vi "Word Wrapping in Picture Control.vi"() -> ()   [LabVIEW 2023]
doc: "This VI takes an array of strings and fades the text in and out of a 2D Picture."
panel:
  in  "Text orientation":T1(ring)
  in  "Text":string[](array[string])=["Demonstrates the use of", "the Draw Text at Point VI", "to draw animated text", "within a 2D Picture."]
  in  "Stop":bool
  out "Picture":picture
  # "Overview: Demonstrates the use of the Draw Text at Point VI to draw animated text within a 2D Picture.\nInstructions: \n1. Run the VI. \n2. Change the Text and Text Orientation values to modify the appearance of the animated text in the Picture indicator.\n3. Click Stop to stop the VI."
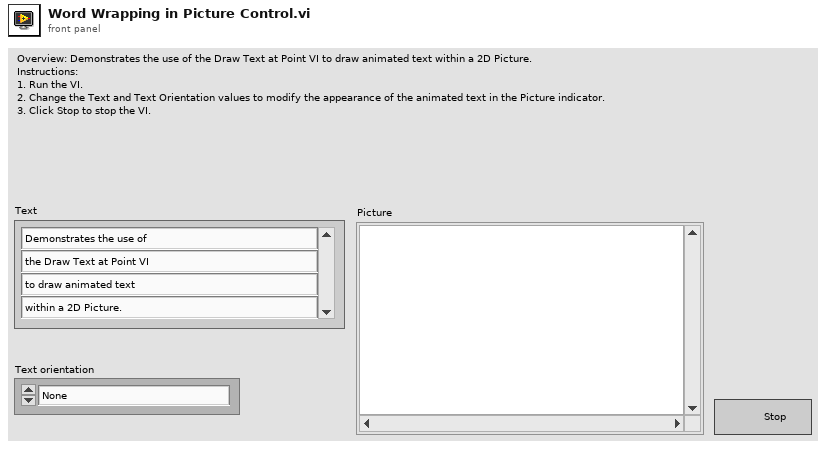
[diagram p1: front panel]
types:
  T1 = enum16{"None", "Stacked", "Clockwise", "Counterclockwise"}
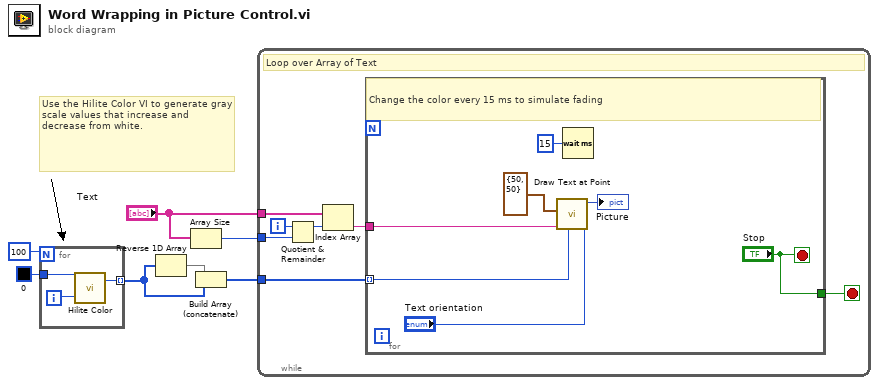
[diagram p0: block diagram]
diagram:
  # "Use the Hilite Color VI to generate gray scale values that increase and decrease from white."
  n1 = for {
    N: 100 -> [_]
    tunnel: u32 0 ("text color(black)") -> [w10]
    tunnel: [w9] -> w4 mode=indexing
    i -> [w8]
    n2 = call <vilib>:"Hilite Color.vi"("Percentage(30)"=w8, "Color In"=w10) -> ("Hilite"=w9:u32)  [unwired: 1 out]
  }
  n3 = Reverse 1D Array(array=w4) -> (reversed array=w5:u32[])
  n4 = Array Size(array="Text") -> (size(s)=w1:i32)
  n5 = Build Array (concatenate)(w5, w4) -> (w3:u32[])
  n6 = while {
    tunnel: "Text" -> [w15]
    tunnel: w3 -> [w17]
    tunnel: w1 -> [w12]
    i -> [w13]
    stop <- w16 stop-if-true
    # "Loop over Array of Text"
    n7 = Quotient & Remainder(x=w13, y=w12) -> (x-y*floor(x/y)=w11:i32)  [unwired: 1 out]
    n8 = Index Array(array=w15, index=w11) -> (element=w14:string)
    n9 = for {
      tunnel: w14 -> [w24]
      tunnel: w17 -> [w23] mode=indexing
      tunnel: ["Stop"] -> w16
      stop <- "Stop" stop-if-true
      # "Change the color every 15 ms to simulate fading"
      n10 = call <vilib>:"Draw Text at Point.vi"("text orientation"="Text orientation", "text color(black)"=w23, "text"=w24, "origin"=cluster{"x":i16, "y":i16} {"x"=50, "y"=50} ("Origin")) -> ("new picture"=→"Picture":picture)  [unwired: 6 in, 1 out]
      n11 = Wait (ms)(milliseconds to wait=u32 15) -> ()  [unwired: 1 out]
    }
  }
